vi "TEST - Force File Move.vi"(8 "error in (no error)":errorcluster) -> (0 "error out":errorcluster, 2 "pass":bool)   [LabVIEW 2020]
uses:
  <userlib>/_OpenG.lib/error/error.llb/openg_error.lvlib
  source/library/openg_file.lvlib
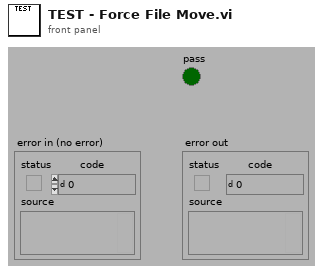
[diagram p1: front panel]
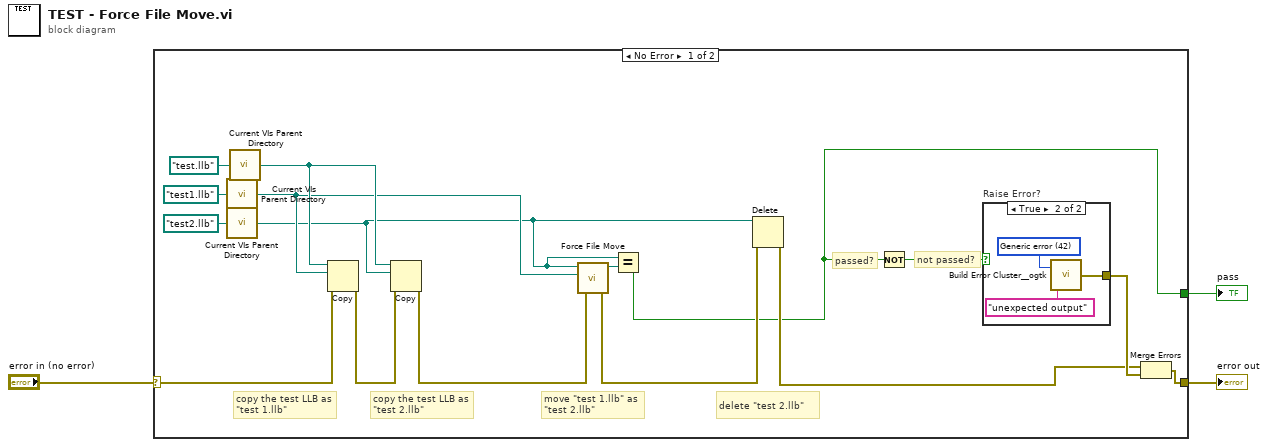
[diagram p0: block diagram]
diagram:
  n1 = case shown="No Error" "error in (no error)" {
    selector: "error in (no error)" -> [w11 w23]
    tunnel: [w4 _] -> w3
    tunnel: [w19 w23] -> w1
    frame No Error {
      # "delete \"test 2.llb\""
      # "move \"test 1.llb\" as \"test 2.llb\""
      # "copy the test LLB as \"test 2.llb\""
      # "copy the test LLB as \"test 1.llb\""
      # "not passed?"
      # "passed?"
      n2 = call "Current VIs Parent Directory.vi"("Relative path (.)"=path "test1.llb") -> ("Parent Directory (+ Relative)"=w6:path)  [unwired: 4 in]
      n3 = call "Current VIs Parent Directory.vi"("Relative path (.)"=path "test2.llb") -> ("Parent Directory (+ Relative)"=w5:path)  [unwired: 4 in]
      n4 = call "Current VIs Parent Directory.vi"("Relative path (.)"=path "test.llb") -> ("Parent Directory (+ Relative)"=w7:path)  [unwired: 4 in]
      n5 = Copy(8:w11, 10:w6, 11:w7) -> (0:w8:errorcluster)  [unwired: 2 in, 2 out]
      n6 = Copy(8:w8, 10:w5, 11:w7) -> (0:w9:errorcluster)  [unwired: 2 in, 2 out]
      n7 = call "Force File Move.vi"("error in (no error)"=w9, "source"=w6, "target"=w5) -> ("error out"=w12:errorcluster, "target out"=w13:path)  [unwired: 3 in]
      n8 = Equal?(x=w5, y=w13) -> (x = y?=w4:bool)
      n9 = Delete(path (use dialog)=w5, error in=w12) -> (error out=w16:errorcluster)  [unwired: 3 in, 2 out]
      n10 = Not(x=w4) -> (.not. x?=w17:bool)
      n11 = case "Raise Error?" shown="True" w17 {
        tunnel: [_ w20] -> w18
        frame False {
        }
        frame True {
          w21 = 42 items=["No error", "Argument error", "Memory is full", "Out of zone", "End of file", "File already open", "Generic file I/O error", "File not found", "File permission error", "Disk is full", "Duplicate path", "Too many files open", "System feature not enabled", "Resource file not found", "Cannot add resource", "Resource not found", "Image not found", "Image memory error", "Pen does not exist", "Config type invalid", "Config token not found", "Config parse error", "Config memory error", "Bad external code format", "Bad external code offset", "External code not present", "Null window", "Destroy window error", "Null menu", "Print aborted", "Bad print record", "Print driver error", "Windows error during printing", "Memory error during printing", "Print dialog error", "Generic print error", "Invalid device refnum", "Device not found", "Device parameter error", "Device unit error", "Cannot open device", "Device call aborted", "Generic error", "Cancelled by user", "Object ID too low", "Object ID too high", "Object not in heap", "Unknown heap", "Unknown object (invalid DefProc)", "Unknown object (DefProc not in table)", "Message out of range", "Invalid (null) method", "Unknown message", "Manager call not supported", "Bad address", "Network operation in progress", "Network operation timed out", "Connection is busy", "Network attribute not supported", "Network error", "Address in use", "System out of memory", "Connection aborted", "Connection refused", "Not connected", "Already connected", "Connection closed", "Initialization error (interapplication manager)", "Bad occurrence", "Wait on unbound occurrence handler", "Occurrence queue overflow", "Datalog type conflict", "Unused", "Unrecognized type (interapplication manager)", "Memory corrupt", "Failed to make temporary DLL", "Old CIN version", "Drag socket not found", "Failed to load drop-object", "Failed to register OLE object", "Failed to release OLE object", "Format specifier type mismatch", "Unknown format specifier", "Too few format specifiers", "Too many format specifiers", "Scan failed", "Newer CIN version", "Error converting to variant", "Runtime menu error", "Password tampered", "Variant attribute not found", "Incompatible variant data type", "Event data is not available", "Event Store is not present", "Occurrence is not found", "Event Queue is not created", "Event info is not available", "Refnum passed is NULL", "Error retrieving Class GUID", "Error retrieving CoClass GUID", "Error retrieving TypeLib GUID.", "Bad built application magic bytes.", "Specific driver is different from the specific driver associated with the Logical Name.", "There is no session opened to the class driver.", "Max Error", "MAX - Error with config objects", "MAX - Error loading configuration", "MAX - Group not supported"]
          n12 = call <userlib>:"Build Error Cluster__ogtk.vi"("String to Prepend to source (\"\")"="unexpected output" ("String to Prepend to source (\"\")"), "code"=w21) -> ("error out"=w20:errorcluster)
        }
      }
      n13 = Merge Errors(w16, w18) -> (w19:errorcluster)
    }
    frame Error {
    }
  }
  "pass" <- w3
  "error out" <- w1
